vi "Add Tag Window.vi"(7 "Database Connection":refnum<k7>, 8 "Error In":errorcluster) -> (0 "Error Out":errorcluster)   [LabVIEW 2019]
uses:
  Controls/Tag Settings.ctl
panel:
  in  "TagData":T1 {"Vmax" min=-10.0 max=10.0 step=1.0; "Vmin" min=-10.0 max=10.0 step=1.0}
  in  "Cancel Button":bool
  in  "OK Button":bool
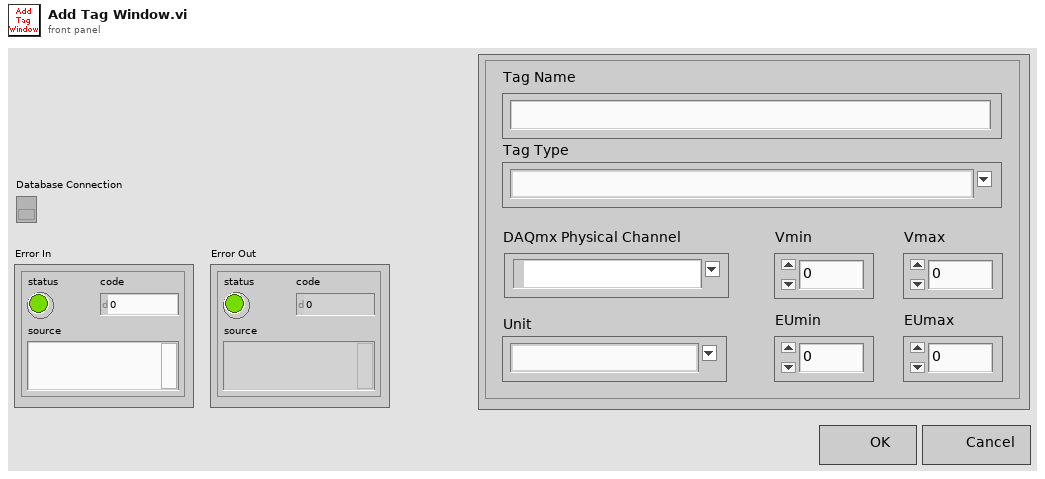
[diagram p1: front panel]
types:
  T1 = typedef "Tag Settings.ctl" = cluster{"Tag Name":string, "Tag Type":string, "DAQmx Physical Channel":tag, "Vmin":dbl, "Vmax":dbl, "Unit":string, "EUmin":dbl, "EUmax":dbl}
  T2 = typedef "Device Settings.ctl" = cluster{"Device Type":string, "Device Name":string, "DAQmx Name":tag, "Terminal Wiring":i32}
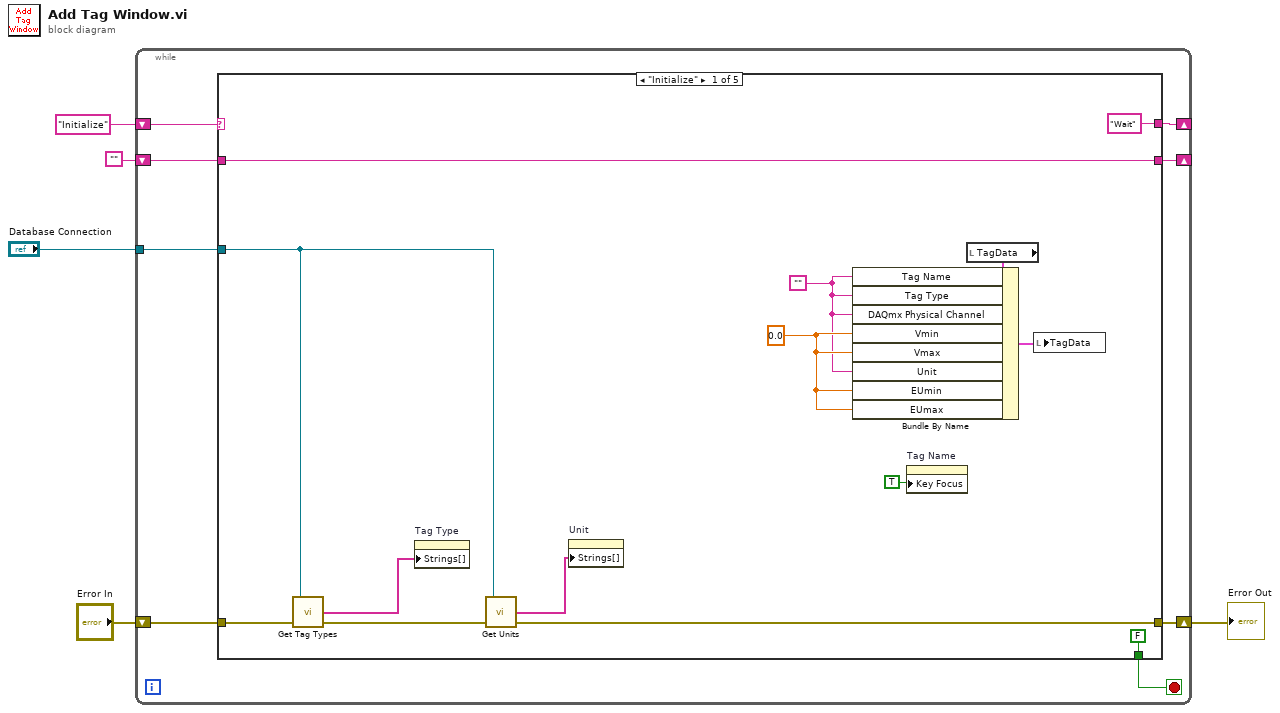
[diagram p0: block diagram]
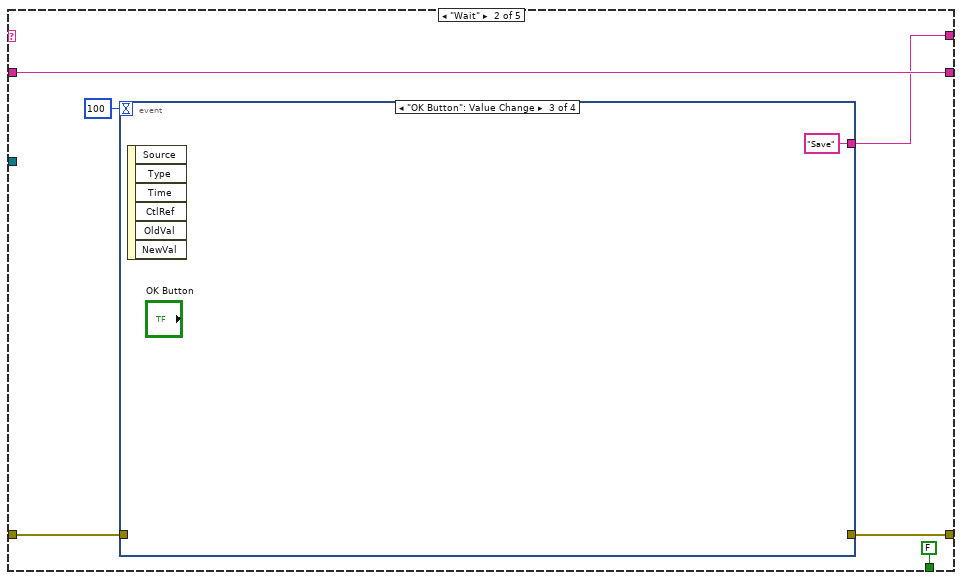
[diagram p2: hidden frame]
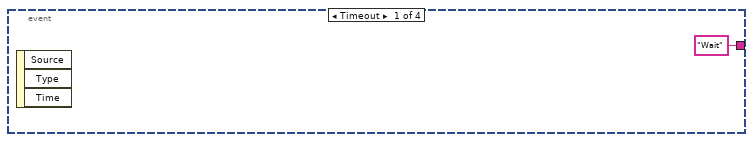
[diagram p3: hidden frame]
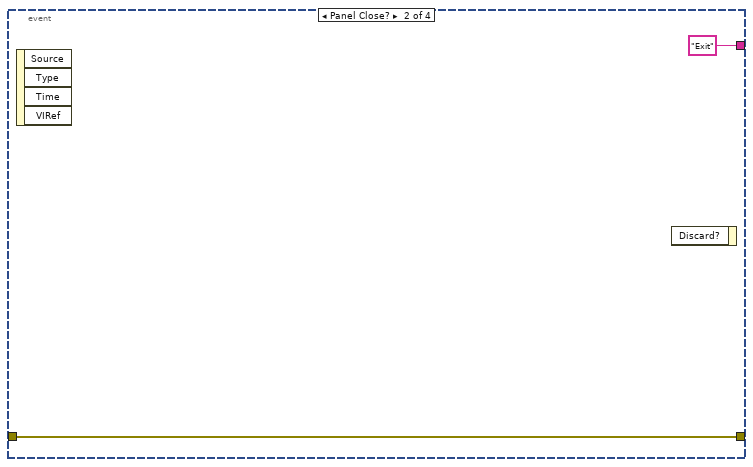
[diagram p4: hidden frame]
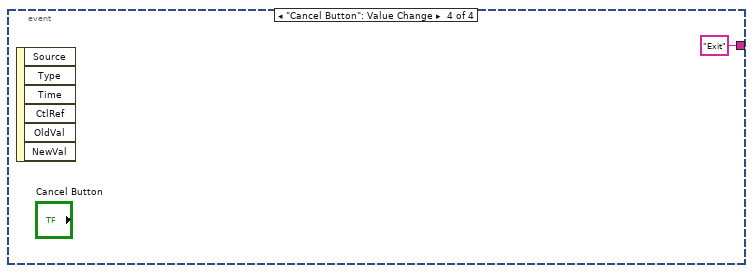
[diagram p5: hidden frame]
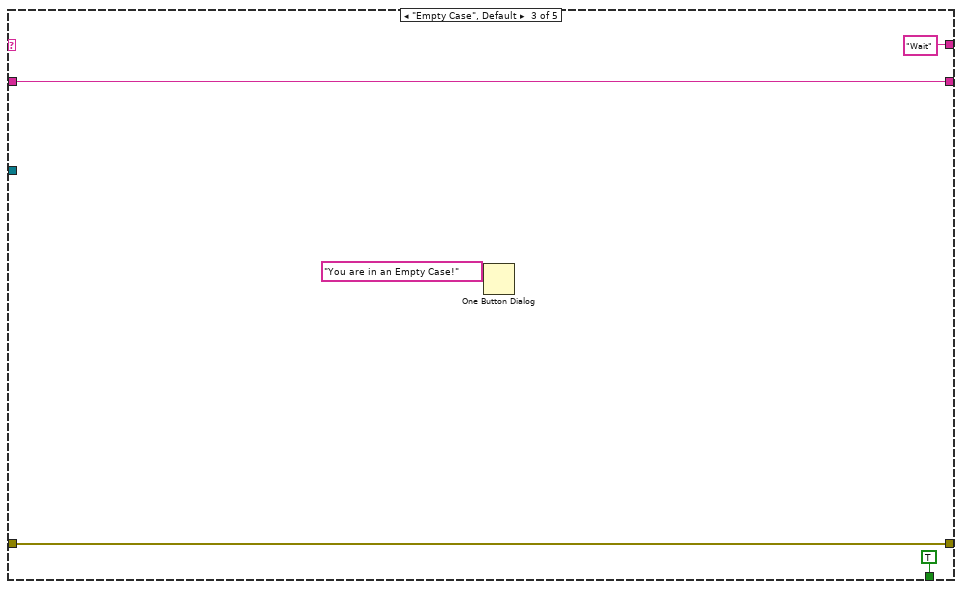
[diagram p6: hidden frame]
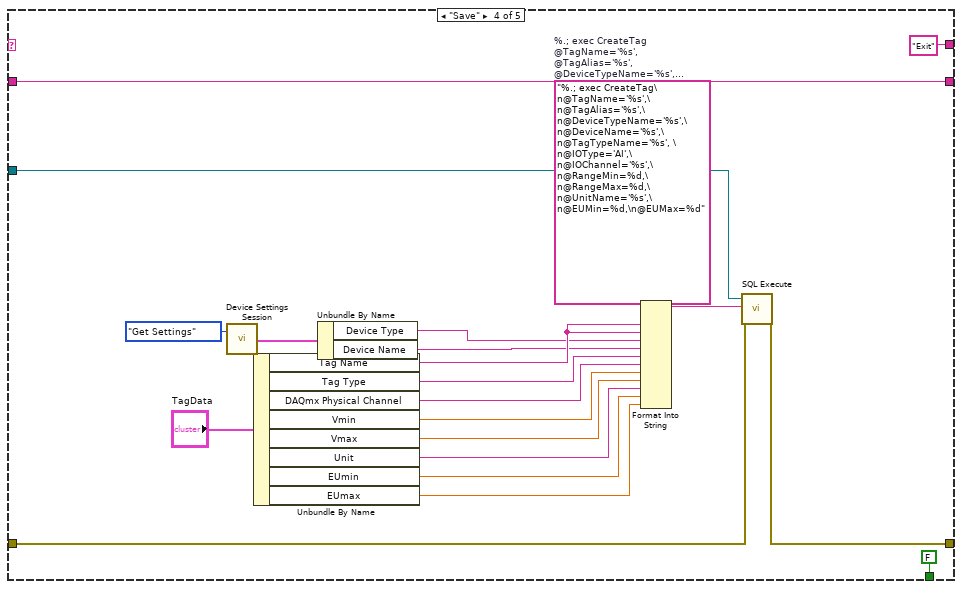
[diagram p7: hidden frame]
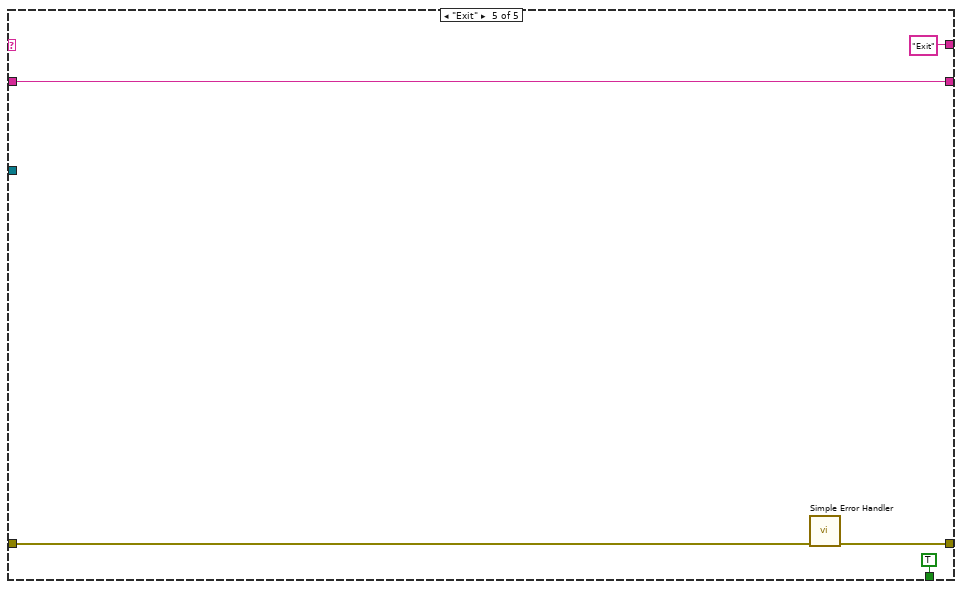
[diagram p8: hidden frame]
diagram:
  n1 = while {
    shift-right: [w9] -> _
    shift-left: "Initialize" ("key") -> [w13]
    shift-right: [w10] -> _
    shift-left: "" -> [w12]
    shift-right: [w7] -> w3
    shift-left: "Error In" -> [w11]
    tunnel: "Database Connection" -> [w6]
    stop <- w8 stop-if-true
    n2 = case shown="\"Initialize\"" w13 {
      tunnel: w12 -> [w25 w32 w40 w62 w69]
      tunnel: w11 -> [w18 w29 w41 w56 w66]
      tunnel: [w25 w32 w40 w62 w69] -> w10
      tunnel: ["Wait" ("key") w31 "Wait" ("key") "Exit" ("key") "Exit" ("key")] -> w9
      tunnel: [FALSE FALSE TRUE FALSE TRUE] -> w8
      tunnel: [w17 w28 w41 w55 w65] -> w7
      tunnel: w6 -> [w16 _ _ w57 _]
      frame "Initialize" {
        w22 = 0.0 ("Vmin")
        w21 = ""
        n3 = call "Get Tag Types.vi"("Error In"=w18, "Database Connection"=w16) -> ("Error Out"=w19:errorcluster, "TagTypeNames"=w15:string[])  [unwired: 1 in, 1 out]
        n4 = property on="Tag Type" class="CmbBox"("Strings[]"=w15) -> ()  [unwired: 2 in, 2 out]
        n5 = call "Get Units.vi"("Error In"=w19, "Database Connection"=w16) -> ("Error Out"=w17:errorcluster, "UnitNames"=w20:string[])  [unwired: 1 in, 1 out]
        n6 = property on="Unit" class="CmbBox"("Strings[]"=w20) -> ()  [unwired: 2 in, 2 out]
        n7 = property on="Tag Name" class="Str"("Key Focus"=TRUE) -> ()  [unwired: 2 in, 2 out]
        n8 = local read "TagData"() -> (w24:T1)
        n9 = Bundle By Name(cluster=w24, "Tag Name"=w21, "Tag Type"=w21, "DAQmx Physical Channel"=w21, "Vmin"=w22, "Vmax"=w22, "Unit"=w21, "EUmin"=w22, "EUmax"=w22) -> (w23:T1)
        n10 = local write "TagData"(w23) -> ()
      }
      frame "Wait" {
        n11 = event shown="[2] \"OK Button\": Value Change" {
          selector: _ -> [_ _ _ _]
          dyn-events: _ -> [_ _ _ _]
          timeout: 100 -> [_ _ _ _]
          tunnel: ["Wait" ("key") "Exit" ("key") "Save" ("key") "Exit" ("key")] -> w31
          tunnel: w29 -> [_ w35 _ _]
          tunnel: [_ w35 _ _] -> w28
          event Timeout {
            n12 = event-data() -> ()  [unwired: 1 in, 3 out]
          }
          event Panel Close? {
            n13 = event-data() -> ()  [unwired: 1 in, 4 out]
            n14 = event-data() -> ()  [unwired: 2 in, 1 out]
          }
          event "OK Button": Value Change {
            n15 = event-data() -> ()  [unwired: 1 in, 6 out]
          }
          event "Cancel Button": Value Change {
            n16 = event-data() -> ()  [unwired: 1 in, 6 out]
          }
        }
      }
      frame "Empty Case", Default {
        n17 = One Button Dialog(message="You are in an Empty Case!") -> ()  [unwired: 1 in, 1 out]
      }
      frame "Save" {
        w60 = "%.; exec CreateTag\n@TagName='%s',\n@TagAlias='%s',\n@DeviceTypeName='%s',\n@DeviceName='%s',\n@TagTypeName='%s', \n@IOType='AI',\n@IOChannel='%s',\n@RangeMin=%d,\n@RangeMax=%d,\n@UnitName='%s',\n@EUMin=%d,\n@EUMax=%d"  # %.; exec CreateTag @TagName='%s', @TagAlias='%s', @DeviceTypeName='%s', @DeviceName='%s', @TagTypeName='%s',  @IOType='AI', @IOChannel='%s', @RangeMin=%d, @RangeMax=%d, @UnitName='%s', @EUMin=%d, @EUMax=%d
        n18 = call "Device Settings Session.vi"("Type"=enum16{"Set Settings", "Get Settings"}."Get Settings") -> ("Device Settings"=w53:T2)  [unwired: 1 in, 1 out]
        n19 = Unbundle By Name("TagData") -> ("Tag Name"=w59:string, "Tag Type"=w50:string, "DAQmx Physical Channel"=w49:tag, "Vmin"=w48:dbl, "Vmax"=w47:dbl, "Unit"=w46:string, "EUmin"=w45:dbl, "EUmax"=w44:dbl)
        n20 = Unbundle By Name(w53) -> ("Device Type"=w52:string, "Device Name"=w51:string)
        n21 = Format Into String(format string=w60, w59, w59, w52, w51, w50, w49, w48, w47, w46, w45, w44) -> (resulting string=w58:string)  [unwired: 2 in, 1 out]
        n22 = call <vilib>:"SQL Execute.vi"("Connection In"=w57, "SQL Query"=w58, "Error in (no error)"=w56) -> ("Error out"=w55:errorcluster)  [unwired: 15 in, 1 out]
      }
      frame "Exit" {
        n23 = call <vilib>:"Simple Error Handler.vi"("error in (no error)"=w66) -> ("error out"=w65:errorcluster)  [unwired: 4 in, 4 out]
      }
    }
  }
  "Error Out" <- w3
